vi "Set ini value.vi"(8 "error in (no error)":errorcluster, 10 "Update values":string[](array[string]), 11 "configuration file path":path=path "C:/UTP/misc/Settings.ini") -> (0 "error out":errorcluster)   [LabVIEW 2023]
uses:
  <vilib>/Utility/config.llb/NI_LVConfig.lvlib
  <vilib>/Utility/config.llb/Write Key (String).vi
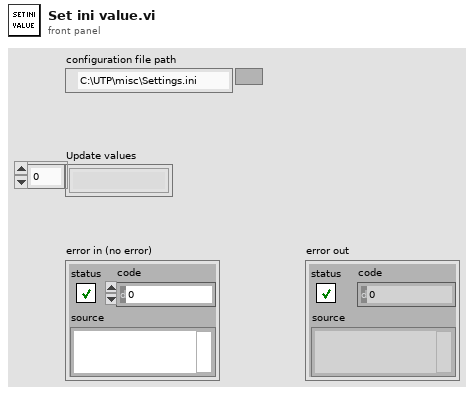
[diagram p1: front panel]
types:
  T1 = typedef "NI_LVConfig.lvlib/Config Data RefNum.ctl" = refnum<k1>
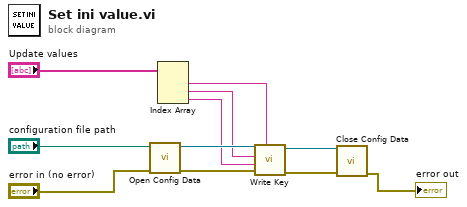
[diagram p0: block diagram]
diagram:
  n1 = call <vilib>:"Open Config Data.vi"("error in (no error)"="error in (no error)", "configuration file path"="configuration file path") -> ("error out"=w7:errorcluster, "refnum"=w8:T1)  [unwired: 7 in, 1 out]
  n2 = Index Array(array="Update values") -> (element #1=w5:string, element #2=w4:string, element #3=w3:string)  [unwired: 3 in]
  n3 = call-poly <vilib>:"Write Key.vi"("section"=w5, "error in (no error)"=w7, "value"=w3, "key"=w4, "refnum"=w8) -> ("error out"=w1:errorcluster, "refnum out"=w2:T1)  [unwired: 4 in, 1 out]
  n4 = call <vilib>:"Close Config Data.vi"("error in (no error)"=w1, "refnum"=w2) -> ("error out"=→"error out":errorcluster)  [unwired: 8 in, 1 out]
